vi "Main.vi"() -> ()   [LabVIEW 2014]
uses:
  BlackPetrol Folder/BlackPetrol.lvclass
panel:
  out "MsgString":string
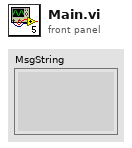
[diagram p1: front panel]
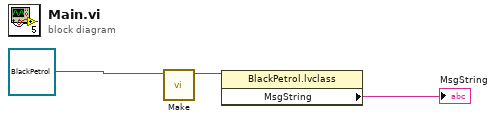
[diagram p0: block diagram]
diagram:
  n1 = call-dynamic "Make.vi"("Electrical in"=refnum<class "BlackPetrol.lvclass"> refnum ("BlackPetrol.lvclass")) -> ("Electrical out"=w3:refnum<class "BlackPetrol.lvclass">)  [unwired: 9 in, 1 out]
  n2 = property class="BlackPetrol.lvclass"(reference=w3) -> ("MsgString"=→"MsgString":string)  [unwired: 1 in, 2 out]
